vi "Scan_step.vi"(0 "Power Supply":refnum<visa-resource-name>, 1 "Exposure Time (s)":dbl format="%#_13g", 2 "Number of Accumulations":i32, 3 "Location of SHG_scat_scan.exe":path, 4 "Location of batch_shg":path, 5 "Error in (Power Supply)":T2, 6 "Location of Take_bck_scan.exe":path, 7 "Max Angle":dbl format="%#_13g", 9 "Min Angle":dbl format="%#_13g", 10 "Location of batch_bck":path, 11 "Angle Resolution":i32, 12 "Stage Connection in":T1, 13 "Error in (Stage)":T2, 14 "Group Name":string, 15 "DataFile name":string) -> ()   [LabVIEW 2017]
uses:
  <instrlib>/Keithley 2200 Series/Keithley 2200 Series.lvlib
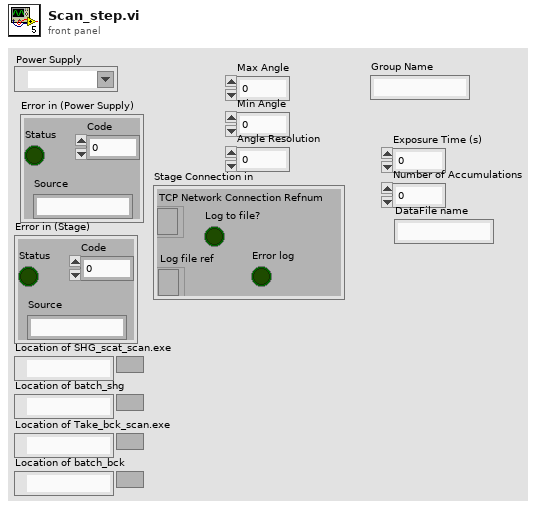
[diagram p1: front panel]
types:
  T1 = cluster{"TCP Network Connection Refnum":refnum<k5>, "Log to file?":bool, "Log file ref":refnum<file>, "Error log":bool}
  T2 = cluster{"Status":bool, "Code":dbl, "Source":string}
  T3 = cluster{"connection TCP":refnum<k5>, "LogTo File":bool, "Log File refnum":refnum<file>, "no error if error log":bool}
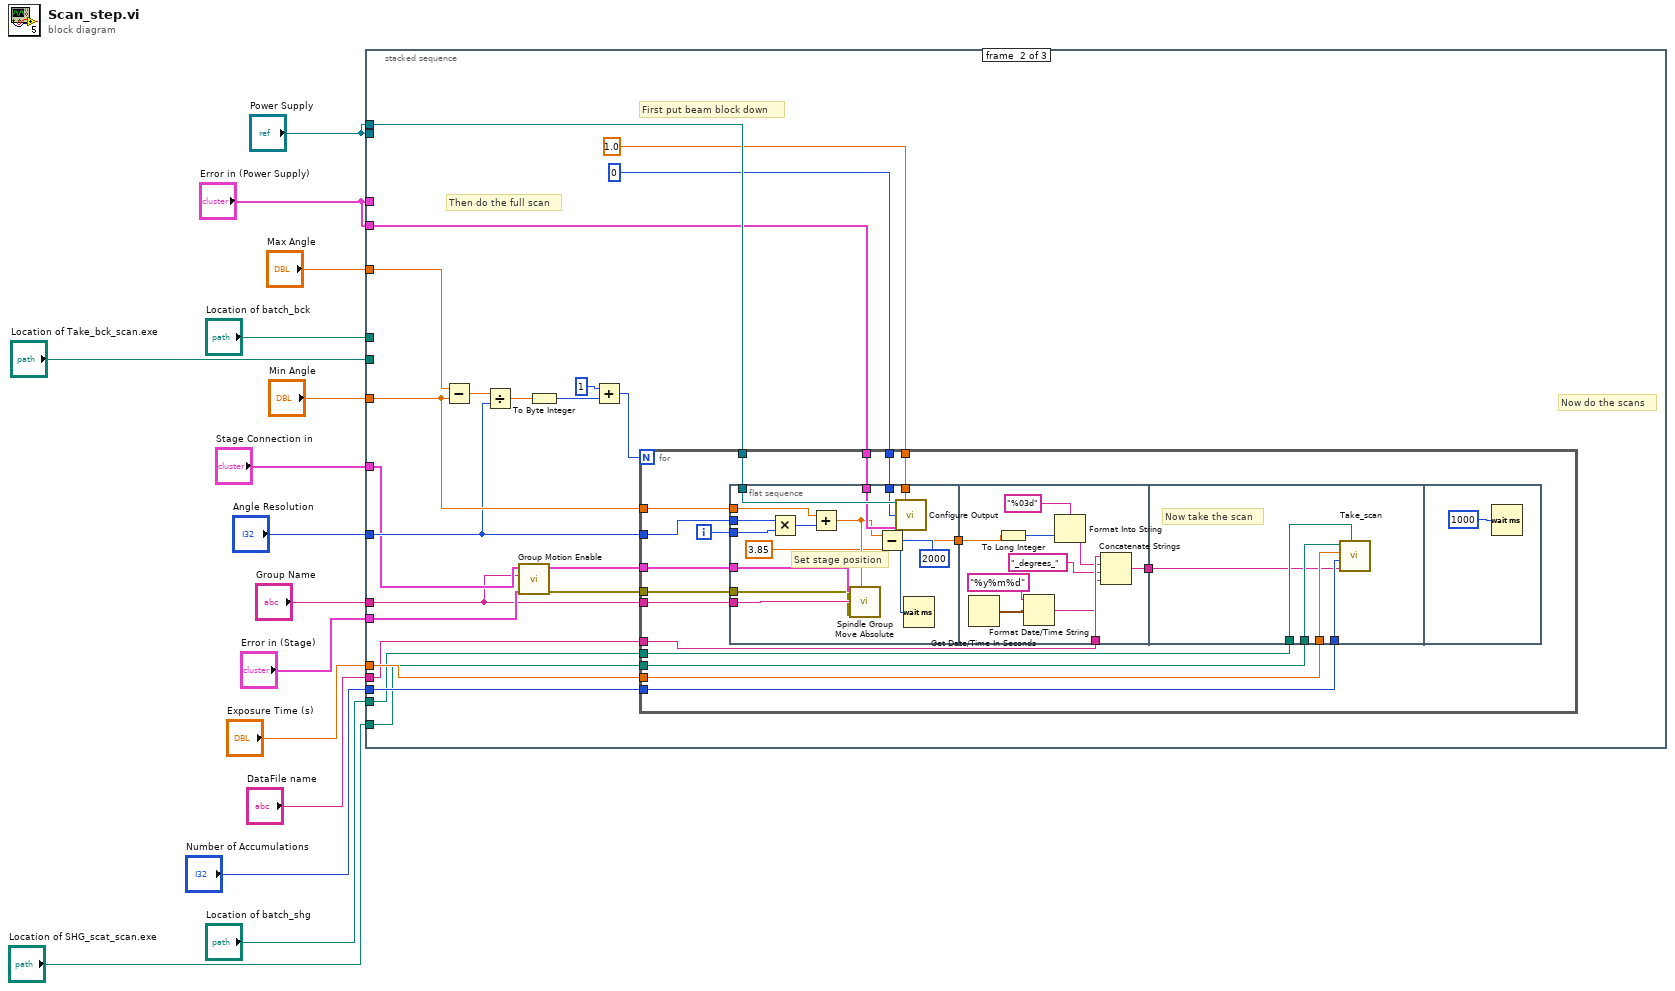
[diagram p0: block diagram]
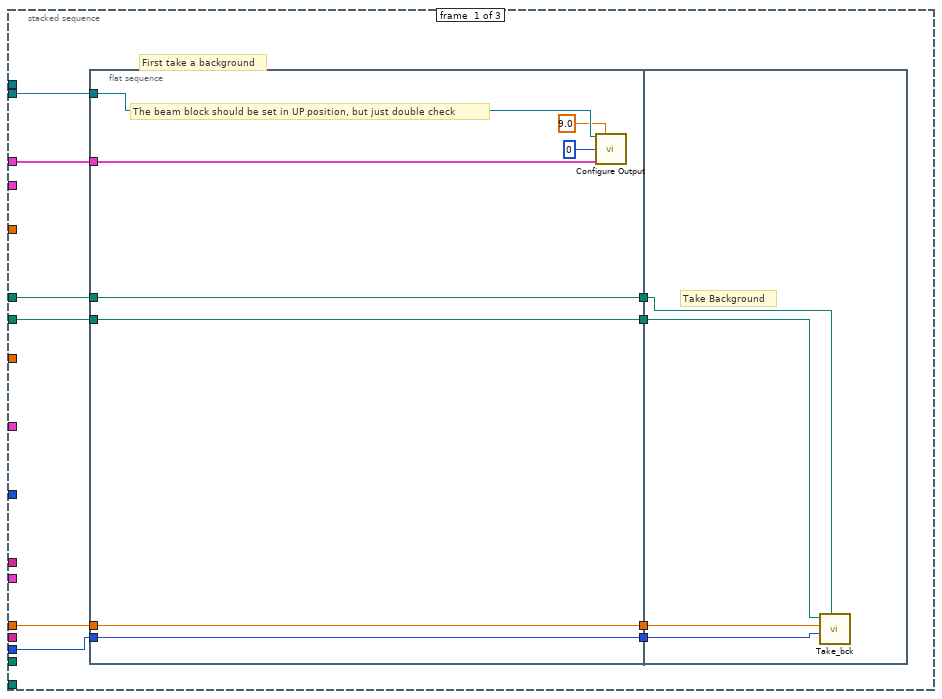
[diagram p2: hidden frame]
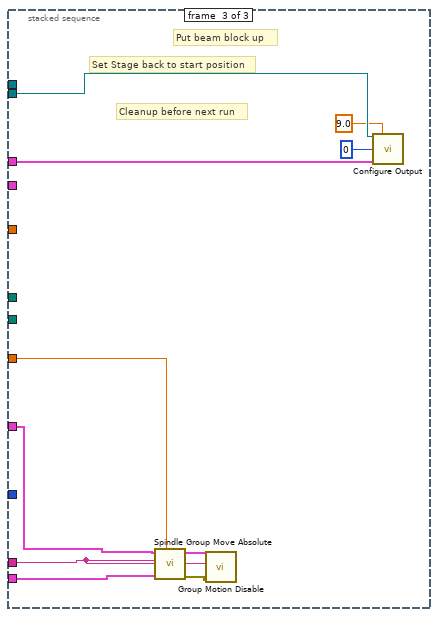
[diagram p3: hidden frame]
diagram:
  n1 = stacked-sequence {
    tunnel: "Power Supply" -> [w24 _ w116]
    tunnel: "Error in (Power Supply)" -> [w25 _ w115]
    tunnel: "Max Angle" -> [_ w59 _]
    tunnel: "Min Angle" -> [_ w56 w114]
    tunnel: "Angle Resolution" -> [_ w55 _]
    tunnel: "Error in (Stage)" -> [_ w45 w108]
    tunnel: "Group Name" -> [_ w44 w110]
    tunnel: "Stage Connection in" -> [_ w46 w109]
    tunnel: "Exposure Time (s)" -> [w23 w51 _]
    tunnel: "Number of Accumulations" -> [w21 w50 _]
    tunnel: "Location of SHG_scat_scan.exe" -> [_ w49 _]
    tunnel: "Location of batch_shg" -> [_ w48 _]
    tunnel: "DataFile name" -> [_ w47 _]
    tunnel: "Location of Take_bck_scan.exe" -> [w19 _ _]
    tunnel: "Location of batch_bck" -> [w17 _ _]
    tunnel: "Power Supply" -> [_ w41 _]
    tunnel: "Error in (Power Supply)" -> [_ w38 _]
    frame #0 {
      # "First take a background"
      n2 = flat-sequence {
        tunnel: w25 -> [w33]
        tunnel: w24 -> [w32]
        tunnel: w23 -> [w30]
        tunnel: [w30] -> w22
        tunnel: w21 -> [w29]
        tunnel: [w29] -> w20
        tunnel: w19 -> [w28]
        tunnel: [w28] -> w18
        tunnel: w17 -> [w27]
        tunnel: [w27] -> w16
        tunnel: w22 -> [w37]
        tunnel: w20 -> [w36]
        tunnel: w18 -> [w35]
        tunnel: w16 -> [w34]
        frame #0 {
          # "The beam block should be set in UP position, but just double check"
          n3 = call <instrlib>:"Configure Output.vi"("VISA resource name"=w32, "Manual Range(0.00)"=9.0, "Function(0:Voltage)"=0, "error in (no error)"=w33) -> ()  [unwired: 10 in, 2 out]
        }
        frame #1 {
          # "Take Background"
          n4 = call "Take_bck.vi"("batch_bck location (should be on Desktop)"=w34, "Number of Accumulations"=w36, "Exposure Time (s)"=w37, "Take_bck_scan.exe location"=w35) -> ()  [unwired: 8 in]
        }
      }
    }
    frame #1 {
      # "Now do the scans"
      # "First put beam block down"
      # "Then do the full scan"
      n5 = Subtract(x=w59, y=w56) -> (x-y=w58:dbl)
      n6 = Divide(x=w58, y=w55) -> (x/y=w57:dbl)
      n7 = call <userlib>:"Group Motion Enable.vi"("error in (no error)"=w45, "Group Name (250 c max)"=w44, "connection ID in"=w46) -> ("error out"=w42:errorcluster, "connection ID out"=w43:T3)  [unwired: 6 in, 1 out]
      n8 = To Byte Integer(number=w57) -> (8bit integer=w54:i8)
      n9 = Add(x=1, y=w54) -> (x+y=w52:i32)
      n10 = for {
        N: w52 -> [_]
        tunnel: w56 -> [w74]
        tunnel: w55 -> [w76]
        tunnel: w44 -> [w73]
        tunnel: w51 -> [w72]
        tunnel: w50 -> [w71]
        tunnel: w49 -> [w70]
        tunnel: w48 -> [w69]
        tunnel: w47 -> [w68]
        tunnel: w43 -> [w66]
        tunnel: w42 -> [w65]
        tunnel: w41 -> [w64]
        tunnel: 1.0 -> [w63]
        tunnel: 0 -> [w62]
        tunnel: w38 -> [w61]
        i -> [w75]
        n11 = flat-sequence {
          tunnel: w76 -> [w91]
          tunnel: w75 -> [w90]
          tunnel: w74 -> [w89]
          tunnel: w73 -> [w88]
          tunnel: w66 -> [w87]
          tunnel: w65 -> [w86]
          tunnel: w64 -> [w84]
          tunnel: w63 -> [w83]
          tunnel: w62 -> [w82]
          tunnel: w61 -> [w81]
          tunnel: [w77] -> w60
          tunnel: w68 -> [w101]
          tunnel: [w98] -> w67
          tunnel: w60 -> [w92]
          tunnel: w72 -> [w106]
          tunnel: w71 -> [w105]
          tunnel: w70 -> [w104]
          tunnel: w69 -> [w103]
          tunnel: w67 -> [w102]
          frame #0 {
            # "Set stage position"
            n12 = Multiply(x=w91, y=w90) -> (x*y=w79:i32)
            n13 = Add(x=w89, y=w79) -> (x+y=w80:dbl)
            n14 = call <userlib>:"Spindle Group Move Absolute.vi"("Target Position (units)"=w80, "error in (no error)"=w86, "Spindle Group  Name (250 c max)"=w88, "connection ID in"=w87) -> ()  [unwired: 5 in, 3 out]
            n15 = Subtract(x=w80, y=3.85) -> (x-y=w77:dbl)
            n16 = call <instrlib>:"Configure Output.vi"("VISA resource name"=w84, "Manual Range(0.00)"=w83, "Function(0:Voltage)"=w82, "error in (no error)"=w81) -> ()  [unwired: 10 in, 2 out]
            n17 = Wait (ms)(milliseconds to wait=2000) -> ()  [unwired: 1 out]
          }
          frame #1 {
            n18 = Get Date/Time In Seconds() -> (seconds since 1Jan1904=w97:timestamp)
            n19 = To Long Integer(number=w92) -> (32bit integer=w93:i32)
            n20 = Format Date/Time String(time format string (%c)="%y%m%d", seconds (now)=w97) -> (date/time string=w95:string)  [unwired: 1 in]
            n21 = Format Into String(format string="%03d", w93) -> (resulting string=w100:string)  [unwired: 2 in, 1 out]
            n22 = Concatenate Strings(w101, w100, "_degrees_", w95) -> (w98:string)
          }
          frame #2 {
            # "Now take the scan"
            n23 = call "Take_scan.vi"("batch_shg location (should be on Desktop)"=w103, "Output File name"=w102, "Number of Accumulations"=w105, "Exposure Time (s)"=w106, "SHG_scat_scan.exe location"=w104) -> ()  [unwired: 7 in]
          }
          frame #3 {
            n24 = Wait (ms)(milliseconds to wait=1000) -> ()  [unwired: 1 out]
          }
        }
      }
    }
    frame #2 {
      # "Set Stage back to start position"
      # "Put beam block up"
      # "Cleanup before next run"
      n25 = call <userlib>:"Spindle Group Move Absolute.vi"("Target Position (units)"=w114, "error in (no error)"=w108, "Spindle Group  Name (250 c max)"=w110, "connection ID in"=w109) -> ("error out"=w111:errorcluster, "connection ID out"=w112:T3)  [unwired: 5 in, 1 out]
      n26 = call <userlib>:"Group Motion Disable.vi"("error in (no error)"=w111, "Group Name (250 c max)"=w110, "connection ID in"=w112) -> ()  [unwired: 6 in, 3 out]
      n27 = call <instrlib>:"Configure Output.vi"("VISA resource name"=w116, "Manual Range(0.00)"=9.0, "Function(0:Voltage)"=0, "error in (no error)"=w115) -> ()  [unwired: 10 in, 2 out]
    }
  }
